vi "Read configuration.vi"(7 "force loading?":bool=TRUE, 8 "error in (no error)":errorcluster, 11 "Murmex in":refnum<class "ExampleClassB.lvclass">) -> (0 "error out":errorcluster, 3 "Murmex out":refnum<class "ExampleClassB.lvclass">)   [LabVIEW 2012, in "ExampleClassB.lvclass"]
doc: "Reads the XML-based configuration file and populates the configuration cluster accordingly. Configuration file name is <component ID>.xml."
uses:
  ExampleClassB.lvclass
  <vilib>/Distrio/Murmex/Murmex/Murmex.lvclass
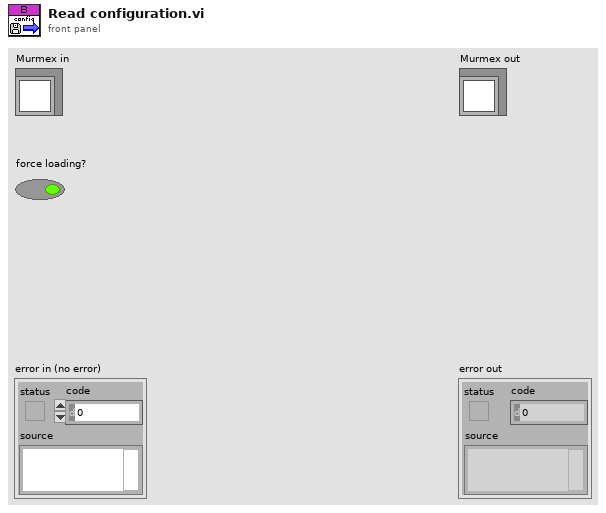
[diagram p1: front panel]
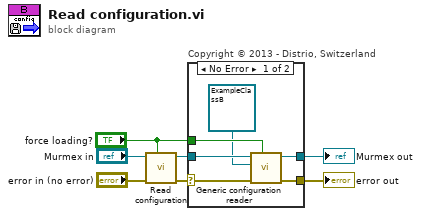
[diagram p0: block diagram]
diagram:
  n1 = call-parent "Read configuration.vi"("force loading?"="force loading?", "error in (no error)"="error in (no error)", "Murmex in"="Murmex in") -> ("error out"=w4:errorcluster, "Murmex out"=w3:refnum<class "ExampleClassB.lvclass">)  [unwired: 7 in]
  n2 = case "Copyright © 2013 - Distrio, Switzerland" shown="No Error" w4 {
    selector: w4 -> [w13 w15]
    tunnel: [w9 w15] -> w1
    tunnel: [w10 w14] -> w2
    tunnel: w3 -> [w11 w14]
    tunnel: "force loading?" -> [w12 _]
    frame No Error {
      n3 = call <vilib>:"Generic configuration reader.vi"("force loading?"=w12, "error in (no error)"=w13, "inheritance level"=refnum<class "ExampleClassB.lvclass"> refnum ("ExampleClassB"), "Murmex in"=w11) -> ("error out"=w9:errorcluster, "Murmex out"=w10:refnum<class "ExampleClassB.lvclass">)  [unwired: 5 in, 1 out]
    }
    frame Error {
    }
  }
  "error out" <- w1
  "Murmex out" <- w2
